vi "Register for Events.vi"(8 "error in (no error)":errorcluster, 11 "2-Axis Stage Status in":refnum<class "2-Axis Stage Status.lvclass">) -> (0 "error out":errorcluster, 2 "Event Refnums":T1, 3 "2-Axis Stage Status out":refnum<class "2-Axis Stage Status.lvclass">)   [LabVIEW 2022 SP3]
uses:
  2-Axis Stage Status.lvclass
  Process Framework/Process State Data/Events.ctl
  Process Framework/Process State Data/Process State Data.lvclass
  XY Controller/XY Stage Data Class/XY Position.ctl
  XY Controller/XY Stage Data Class/XY Stage Data Class.lvclass
  XY Controller/XY Stage Data Class/Moving.ctl
  XY Controller/XY Stage Data Class/Homed.ctl
  XY Controller/XY Stage Data Class/Acceleration.ctl
  XY Controller/XY Stage Data Class/Current Speed.ctl
  XY Controller/XY Stage Data Class/Events.ctl
  XY Controller/XY Stage Data Class/Speed.ctl
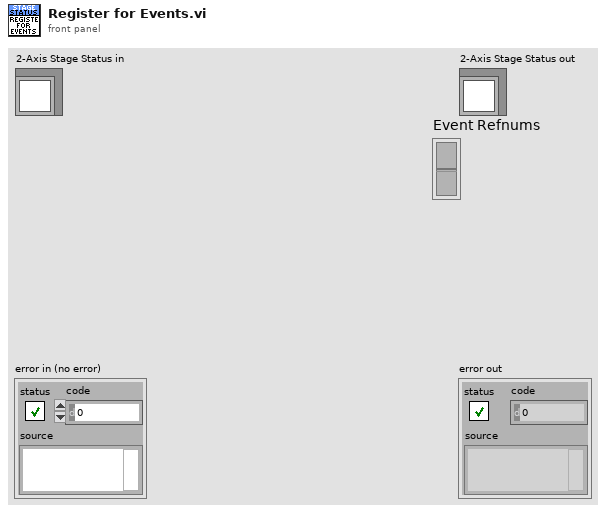
[diagram p1: front panel]
types:
  T1 = cluster{"Event Registration Refnum":refnum<event-registration>, "Event Registration Refnum":refnum<event-registration>}
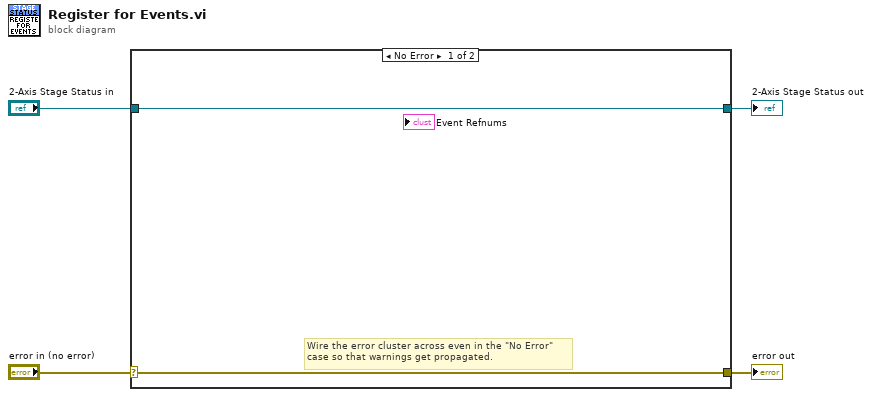
[diagram p0: block diagram]
diagram:
  n1 = case shown="No Error" "error in (no error)" {
    selector: "error in (no error)" -> [w5 w8]
    tunnel: [w5 w8] -> w3
    tunnel: [w6 w7] -> w1
    tunnel: "2-Axis Stage Status in" -> [w6 w7]
    frame No Error {
      # "Wire the error cluster across even in the \"No Error\"\ncase so that warnings get propagated."
    }
    frame Error {
    }
  }
  "error out" <- w3
  "2-Axis Stage Status out" <- w1
